vi "GV_GetEngUnit2.vi"(8 "error in (no error)":errorcluster, 10 "Plot":i32, 11 "TAGproperties":T1 {"TAGprop"."TagFunc" format="%08x"; "TAGprop"."RangeL" format="%.2f"; "TAGprop"."RangeH" format="%.2f"}) -> (0 "error out":errorcluster, 1 "Unit":string)   [LabVIEW 2020, in "Sgraph_lib_V1.lvlib" / "Gviewer.lvclass"]
doc: "Get the engineering unit of a selected trace\n(from Properties Array)"
uses:
  Gviewer.lvclass
  DBAL/controls/DBAL_TAGprops.ctl
  DBAL/controls/DBAL_TAGpropEdit.ctl
  Common/controls/typedef_com_TagProp.ctl
  Builds/Sgraph_lib_V1.lvlib
  DBAL/DBAL.lvclass
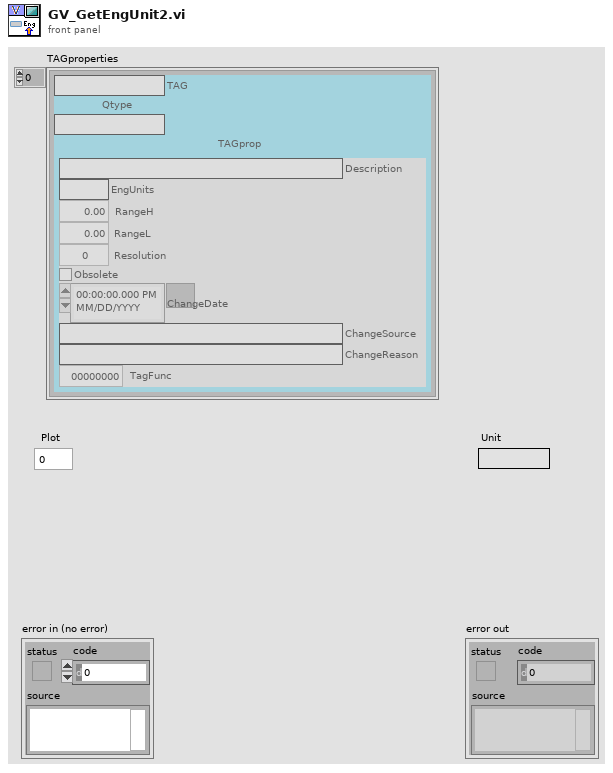
[diagram p1: front panel]
types:
  T1 = typedef "Sgraph_lib_V1.lvlib/DBAL.lvclass/DBAL_TAGprops.ctl" = T2[]
  T2 = typedef "Sgraph_lib_V1.lvlib/DBAL.lvclass/DBAL_TAGpropEdit.ctl" = cluster{"TAG":string, "Qtype":string, "TAGprop":T3}
  T3 = typedef "Sgraph_lib_V1.lvlib/typedef_com_TagProp.ctl" = cluster{"Description":string, "EngUnits":string, "RangeH":dbl, "RangeL":dbl, "Resolution":i32, "Obsolete":bool, "ChangeDate":timestamp, "ChangeSource":string, "ChangeReason":string, "TagFunc":u32}
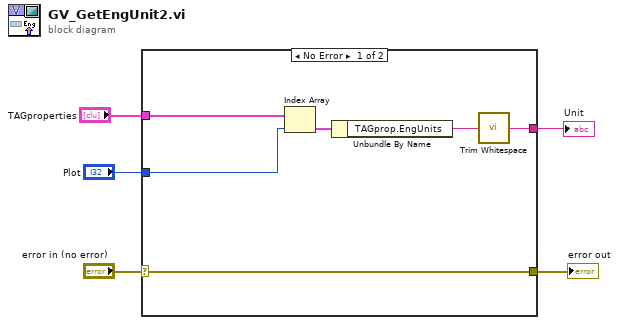
[diagram p0: block diagram]
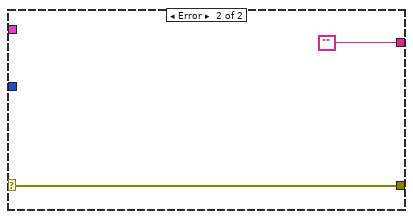
[diagram p2: hidden frame]
diagram:
  n1 = case shown="No Error" "error in (no error)" {
    selector: "error in (no error)" -> [w11 w13]
    tunnel: [w11 w13] -> w4
    tunnel: "Plot" -> [w10 _]
    tunnel: [w7 ""] -> w2
    tunnel: "TAGproperties" -> [w6 _]
    frame No Error {
      n2 = Index Array(array=w6, index=w10) -> (element=w9:T2)
      n3 = Unbundle By Name(w9) -> ("TAGprop.EngUnits"=w8:string)
      n4 = call <vilib>:"Trim Whitespace.vi"("string"=w8) -> ("trimmed string"=w7:string)  [unwired: 1 in]
    }
    frame Error {
    }
  }
  "error out" <- w4
  "Unit" <- w2
